vi "PSRR.vi"() -> ()   [LabVIEW 2020]
uses:
  pmbus_ltm4676a/controls/ltm4676a_config.ctl
  controls/psrr_nightwing_config.ctl
  controls/psrr_heatwave_config.ctl
  controls/psrr_scope_config.ctl
  controls/psrr_fgen_sweep_config.ctl
  <instrlib>/niDCPower/nidcpower.llb/niDCPower Source Mode.ctl
  <instrlib>/niDCPower/nidcpower.llb/niDCPower Output Function.ctl
  <instrlib>/niDCPower/nidcpower.llb/niDCPower Sense.ctl
  <instrlib>/niDCPower/nidcpower.llb/niDCPower Wait For Event - Event.ctl
  <instrlib>/niFgen/niFgen.llb/niFgen Output Mode.ctl
  <instrlib>/niScope/Controls/niScope vertical coupling.ctl
  <instrlib>/niScope/Controls/niScope trigger slope.ctl
  <instrlib>/niScope/Controls/niScope trigger coupling.ctl
  <instrlib>/niScope/Controls/niScope trigger source.ctl
  <instrlib>/niScope/Utility/niScope Get Channel Name From String.vi
  <instrlib>/niScope/Configure/Trigger/niScope Configure Trigger Edge.vi
panel:
  in  "App control":enum32{"Main", "Debug", "Ref"}(tab)
  in  "Calculation method":enum16{"RMS", "Peak-to-peak"}(ring)
  in  "Stop":bool
  in  "Step delay (ms)":u32=50
  in  "Continue sweep":bool
  in  "Step mode":enum16{"Timed", "User"}(ring)
  in  "Config control":T1(tab)
  in  "Source config":T2={"Source device name"="Nightwing", "Source device channel"="0", "Source device voltage (V)"=18.0, "Source current limit (A)"=6.0, "Channel setup time (s)"=0.5} {"Channel setup time (s)" format="%_4p"}
  in  "Load config":T3={"Load device name"="Heat-Wave", "Load device channel"="0", "Load device current (A)"=1.0, "Load voltage limit (V)"=6.0, "Channel setup time (s)"=0.5} {"Channel setup time (s)" format="%_4p"}
  in  "FGEN/sweep config":T4={"FGEN Resource Name"="Dev1", "Channel"="0", "Standard Waveform"=0, "Amplitude"=0.05, "Load impedance"=10000.0, "Sweep type"=1, "Points or Points/Decade"=10, "Start frequency"=10.0, "Stop frequency"=1000000.0} {"Load impedance" min=0.0 step=1000.0 format="%.2p"; "Stop frequency" min=0.0 step=1000.0 format="%.2p"; "Start frequency" min=0.0 step=1000.0 format="%.2p"; "Points or Points/Decade" min=1 step=1; "Sweep type" items=["Linear", "Logarithmic"]; "Amplitude" format="%.2p"; "Standard Waveform" items=["Sine", "Square", "Triangle", "Ramp Up", "Ramp Down", "DC", "Noise"]}
  in  "Scope config":T5={"Resource name"="Dev1", "Scope channel(s)"="0,1", "Probe Attenuation"=10.0, "Samples per cycle"=1000, "Cycles to acquire"=4} {"Cycles to acquire" min=1 step=1; "Probe Attenuation" format="%.1f"; "Samples per cycle" step=1000000}
  in  "LTM4676A Runtime Config":T6={"SDC config path"=path "C:/Users/Administrator/Documents/qkocian-sandbox/demos/argus-buck-demo/instrumentstudio/sdc/pmbus_ltm4676a.sdconfig", "Output setpoint (V)"=3.3, "Voltage margin (%)"=5.0, "Voltage warn limit (%)"=7.5, "Voltage fault limit (%)"=10.0, "Switching frequency (kHz)"=650} {"Switching frequency (kHz)" items=["250"=62440, "350"=64188, "425"=64338, "500"=64488, "575"=575, "650"=650, "750"=750, "1000"=1000]; "Voltage fault limit (%)" min=0.0 max=100.0 step=1.0 format="%.1g"; "Voltage warn limit (%)" min=0.0 max=100.0 step=1.0 format="%.1g"; "Voltage margin (%)" min=0.0 max=100.0 step=1.0 format="%.1g"; "Output setpoint (V)" min=0.5 max=5.5 step=0.1}
  out "Power Supply Rejection Ratio (dB)":cluster{dbl[], dbl[]}(graph) caption="Current (Amps) vs Voltage (Volts)"
  in  "Continue sweep (debug)":bool
  out "Output spectrum(s)":T7(graph)
  out "success?":bool
  in  "Use PMBus?":bool
  out "Input waveform(s)":waveform(dbl)[](graph)
  out "Filtered waveform(s)":waveform(dbl)[](graph) caption="Output waveform(s)"
  out "Detected frequencies":dbl[](array[numeric])
  out "Detected amplitudes":dbl[](array[numeric])
  out "Detected phases (deg)":dbl[](array[numeric])
  out "Actual sample rate":dbl=10000000.0 format="%#.2p"
  out "Actual record length":i32=1000
  out "Reqested sample rate":dbl
  out "Requested record length":i32
  out "Supply voltage":dbl[](array[numeric])
  out "Supply current":dbl[](array[numeric])
  out "Load voltage":dbl[](array[numeric])
  out "Load current":dbl[](array[numeric])
  out "Sweep values":dbl[](array[numeric]) format="%_6g"
  out "PSRR array":dbl[](array[numeric])
  # "(only for Step mode = Timed)"
  # "(only for Step mode = User)"
  # "(only for Step mode = User)"
  # "J2120A Information"
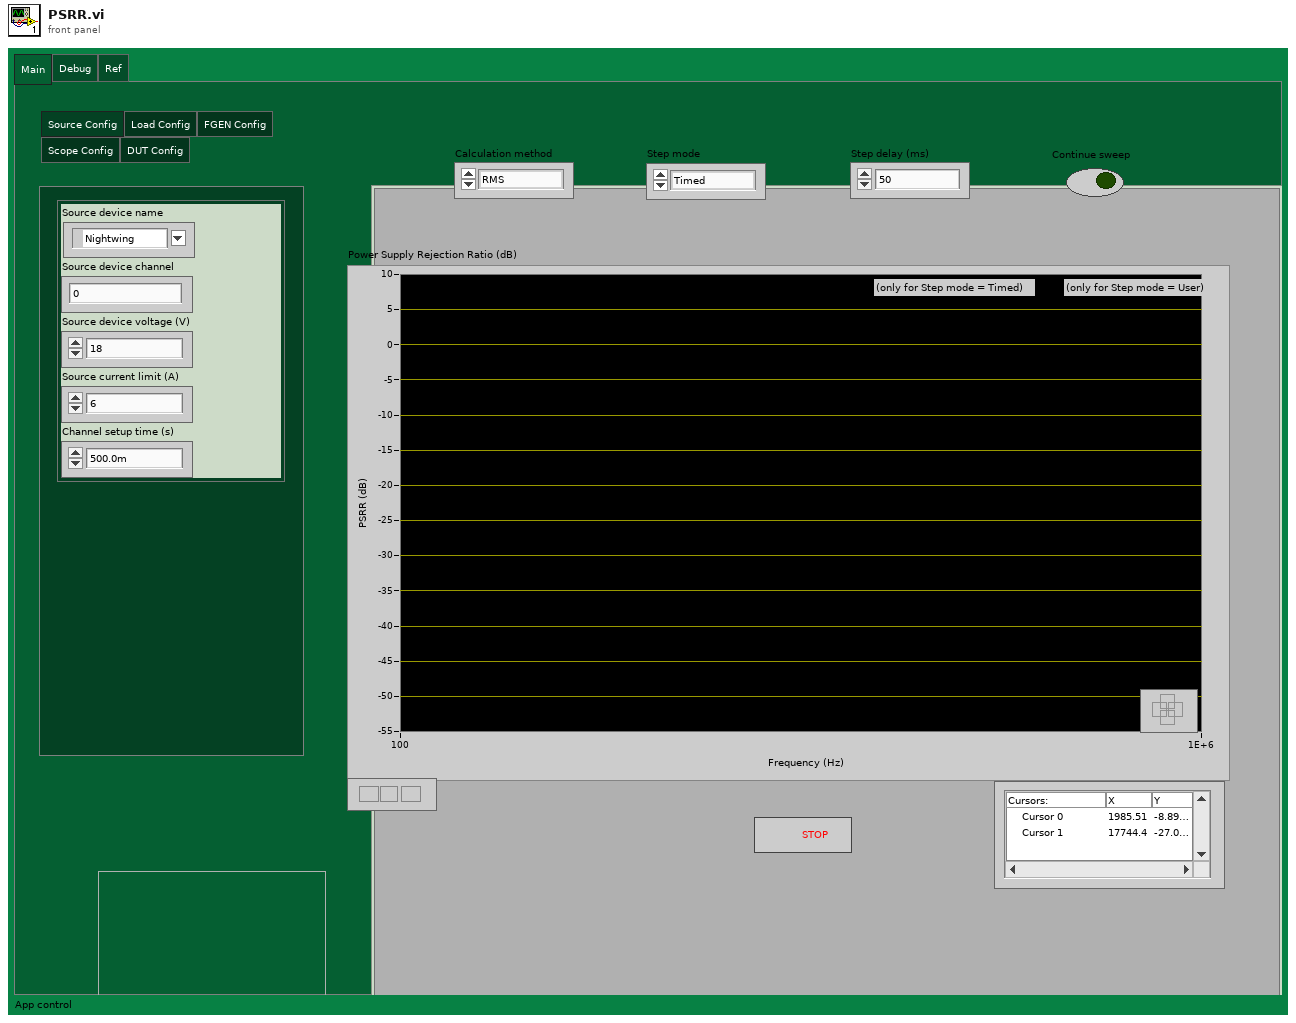
[diagram p1: front panel]
types:
  T1 = enum32{"Source Config", "Load Config", "FGEN Config", "Scope Config", "DUT Config"}
  T2 = typedef "psrr_nightwing_config.ctl" = cluster{"Source device name":refnum<k15>, "Source device channel":string, "Source device voltage (V)":dbl, "Source current limit (A)":dbl, "Channel setup time (s)":dbl}
  T3 = typedef "psrr_heatwave_config.ctl" = cluster{"Load device name":refnum<k15>, "Load device channel":string, "Load device current (A)":dbl, "Load voltage limit (V)":dbl, "Channel setup time (s)":dbl}
  T4 = typedef "psrr_fgen_sweep_config.ctl" = cluster{"FGEN Resource Name":refnum<k15>, "Channel":string, "Standard Waveform":u16, "Amplitude":dbl, "Load impedance":dbl, "Sweep type":u16, "Points or Points/Decade":u16, "Start frequency":dbl, "Stop frequency":dbl}
  T5 = typedef "psrr_scope_config.ctl" = cluster{"Resource name":refnum<k15>, "Scope channel(s)":string, "Probe Attenuation":dbl, "Samples per cycle":u32, "Cycles to acquire":u16}
  T6 = typedef "ltm4676a_config.ctl" = cluster{"SDC config path":path, "Output setpoint (V)":dbl, "Voltage margin (%)":dbl, "Voltage warn limit (%)":dbl, "Voltage fault limit (%)":dbl, "Switching frequency (kHz)":u16}
  T7 = cluster{"f0":dbl, "df":dbl, "dB Spectrum (Hann)":dbl[]}[]
  T8 = typedef "niDCPower Wait For Event - Event.ctl" = i32
  T9 = typedef "niDCPower Sense.ctl" = i32
  T10 = typedef "niDCPower Output Function.ctl" = i32
  T11 = typedef "niDCPower Source Mode.ctl" = i32
  T12 = typedef "niScope trigger source.ctl" = string
  T13 = typedef "niScope trigger coupling.ctl" = u16
  T14 = typedef "niScope trigger slope.ctl" = i32
  T15 = typedef "niScope vertical coupling.ctl" = i32
  T16 = typedef "niFgen Output Mode.ctl" = u32
  T17 = cluster{"Detected frequencies":dbl[], "Detected amplitudes":dbl[], "Detected phases (deg)":dbl[]}
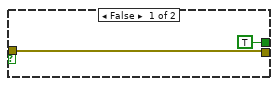
[diagram p2: hidden frame]
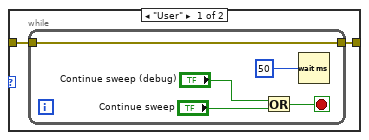
[diagram p4: hidden frame]
diagram:
  w8 = T8 1030 items=["Source Complete Event"=1030, "Measure Complete Event"=1031, "Sequence Iteration Complete Event"=1032, "Sequence Engine Done Event"=1033, "Pulse Complete Event"=1051, "Ready For Pulse Trigger Event"=1052] ("event")
  w31 = 1042 items=["Slow"=1041, "Normal"=1038, "Fast"=1039, "Custom"=1042] ("Source:Transient Response")
  w38 = T9 1008 items=["Local"=1008, "Remote"=1009] ("sense")
  w41 = 1026 items=["Automatically after Source Complete"=1025, "On Demand"=1026, "On Measure Trigger"=1027] ("Measurement:Advanced:Measure When")
  w50 = 1 items=["Off", "On"] ("Source:DC Voltage:Current Limit Autorange")
  w52 = T10 1006 items=["DC Voltage"=1006, "DC Current"=1007, "Pulse Voltage"=1049, "Pulse Current"=1050] ("output function")
  w55 = T11 1020 items=["Single Point"=1020, "Sequence"=1021] ("source mode")
  n1 = Unbundle By Name("Source config") -> ("Source device channel"=w1:string, "Source device name"=w29:refnum<k15>)
  n2 = call <instrlib>:"niDCPower Initialize With Independent Channels.vi"("resource name"=w29) -> ("error out"=w39:errorcluster, "instrument handle out"=w40:refnum<k15>)  [unwired: 9 in]
  n3 = call <instrlib>:"niDCPower Configure Sense.vi"("error in (no error)"=w39, "sense"=w38, "channel name"=w1, "instrument handle"=w40) -> ("error out"=w28:errorcluster, "instrument handle out"=w27:refnum<k15>)  [unwired: 6 in]
  n4 = call <instrlib>:"niDCPower Configure Source Mode With Channels.vi"("error in (no error)"=w28, "source mode"=w55, "channel name"=w1, "instrument handle"=w27) -> ("error out"=w54:errorcluster, "instrument handle out"=w53:refnum<k15>)  [unwired: 6 in]
  n5 = Unbundle By Name("Source config") -> ("Source device voltage (V)"=w13:dbl, "Source current limit (A)"=w14:dbl, "Channel setup time (s)"=w12:dbl)
  n6 = call <instrlib>:"niDCPower Configure Output Function.vi"("error in (no error)"=w54, "output function"=w52, "channel name"=w1, "instrument handle"=w53) -> ("error out"=w45:errorcluster, "instrument handle out"=w44:refnum<k15>)  [unwired: 6 in]
  n7 = call <instrlib>:"niDCPower Configure Voltage Level.vi"("error in (no error)"=w45, "voltage level"=w13, "channel name"=w1, "instrument handle"=w44) -> ("error out"=w42:errorcluster, "instrument handle out"=w43:refnum<k15>)  [unwired: 6 in]
  n8 = call <instrlib>:"niDCPower Configure Current Limit.vi"("error in (no error)"=w42, "current limit"=w14, "channel name"=w1, "instrument handle"=w43) -> ("error out"=w51:errorcluster, "instrument handle out"=w49:refnum<k15>)  [unwired: 6 in]
  n9 = property class="niDCPower"(reference=w49, error in=w51, "Active Channel"=w1, "Voltage Level Autorange"=w50, "Current Limit Autorange"=w50, "Source Delay"=w12, "Measure When"=w41) -> (reference out=w35:refnum<k15>, error out=w34:errorcluster)
  n10 = property class="niDCPower"(reference=w35, error in=w34, "Active Channel"=w1, "Transient Response"=w31, "Voltage GBW"=1000.0 ("Source:Custom Transient Response:Voltage:Gain Bandwidth"), "Voltage Compensation Freq"=1000.0 ("Source:Custom Transient Response:Voltage:Compensation Frequency"), "Voltage Pole-Zero Ratio"=1.0 ("Source:Custom Transient Response:Voltage:Pole-Zero Ratio"), "Current GBW"=1000000.0 ("Source:Custom Transient Response:Current:Gain Bandwidth")) -> (reference out=w33:refnum<k15>, error out=w32:errorcluster)
  n11 = call <instrlib>:"niDCPower Commit With Channels.vi"("error in (no error)"=w32, "channel name"=w1, "instrument handle"=w33) -> ("error out"=w36:errorcluster, "instrument handle out"=w37:refnum<k15>)  [unwired: 7 in]
  n12 = call <instrlib>:"niDCPower Initiate With Channels.vi"("error in (no error)"=w36, "channel name"=w1, "instrument handle"=w37) -> ("error out"=w9:errorcluster, "instrument handle out"=w10:refnum<k15>)  [unwired: 7 in]
  n13 = call <instrlib>:"niDCPower Wait For Event With Channels.vi"("error in (no error)"=w9, "event"=w8, "channel name"=w1, "instrument handle"=w10) -> ("error out"=w7:errorcluster, "instrument handle out"=w6:refnum<k15>)  [unwired: 6 in]
  n14 = call <instrlib>:"niDCPower Measure Multiple.vi"("error in (no error)"=w7, "channel name"=w1, "instrument handle"=w6) -> ("error out"=w5:errorcluster, "current measurements"=→"Supply current":dbl[], "voltage measurements"=→"Supply voltage":dbl[], "instrument handle out"=w4:refnum<k15>)  [unwired: 5 in]
  n15 = case shown="True" "Use PMBus?" {
    tunnel: [w57 w61] -> w26
    tunnel: w5 -> [w57 w60]
    tunnel: [TRUE ("success?") w58] -> w22
    frame False {
    }
    frame True {
      n16 = call "ltm4676a_set_runtime_config.vi"("LTM4676A Runtime Config"="LTM4676A Runtime Config", "error in (no error)"=w60) -> ("success?"=w58:bool, "error out"=w61:errorcluster)  [unwired: 1 out]
      "success?" <- w58
    }
  }
  n17 = case shown="True" w22 {
    tunnel: w26 -> [w62 w178]
    tunnel: [w62 w106] -> w11
    tunnel: w4 -> [w64 w74]
    tunnel: [w64 w72] -> w21
    tunnel: w1 -> [w63 w73]
    tunnel: [w63 w71] -> w20
    frame False {
    }
    frame True {
      w86 = T10 1007 items=["DC Voltage"=1006, "DC Current"=1007, "Pulse Voltage"=1049, "Pulse Current"=1050] ("output function")
      w87 = T11 1020 items=["Single Point"=1020, "Sequence"=1021] ("source mode")
      w89 = 1026 items=["Automatically after Source Complete"=1025, "On Demand"=1026, "On Measure Trigger"=1027] ("Measurement:Advanced:Measure When")
      w134 = 1 items=["None"=1, "Auto Trigger"=2] ("Triggering:Trigger Modifier")
      w141 = T13 1 items=["AC"=0, "DC"=1, "HF Reject"=3, "LF Reject"=4, "AC Plus HF Reject"=1001] ("trigger coupling")
      w142 = T14 0 items=["Positive", "Negative"] ("trigger slope")
      w145 = T15 0 items=["AC", "DC", "Ground"] ("vertical coupling")
      w148 = u32 0 items=["1 mega ohm"=0, "50 ohms"=2] ("input impedance")
      w159 = T16 0 items=["Standard Function", "Frequency List", "Arbitrary Waveform", "Arbitrary Sequence", "Script"] ("Output Mode (default: 0=Standard Function)")
      w90 = 1 items=["Off", "On"] ("Source:DC Current:Current Level Autorange")
      w181 = 1042 items=["Slow"=1041, "Normal"=1038, "Fast"=1039, "Custom"=1042] ("Source:Transient Response")
      w184 = T8 1030 items=["Source Complete Event"=1030, "Measure Complete Event"=1031, "Sequence Iteration Complete Event"=1032, "Sequence Engine Done Event"=1033, "Pulse Complete Event"=1051, "Ready For Pulse Trigger Event"=1052] ("event")
      w187 = T9 1009 items=["Local"=1008, "Remote"=1009] ("sense")
      n18 = Unbundle By Name("Load config") -> ("Load device channel"=w69:string, "Load device name"=w179:refnum<k15>)
      n19 = call <instrlib>:"niDCPower Initialize With Independent Channels.vi"("error in (no error)"=w178, "resource name"=w179) -> ("error out"=w189:errorcluster, "instrument handle out"=w188:refnum<k15>)  [unwired: 8 in]
      n20 = call <instrlib>:"niDCPower Configure Sense.vi"("error in (no error)"=w189, "sense"=w187, "channel name"=w69, "instrument handle"=w188) -> ("error out"=w93:errorcluster, "instrument handle out"=w96:refnum<k15>)  [unwired: 6 in]
      n21 = Unbundle By Name("Load config") -> ("Load device current (A)"=w88:dbl, "Load voltage limit (V)"=w65:dbl, "Channel setup time (s)"=w172:dbl)
      n22 = call <instrlib>:"niDCPower Configure Source Mode With Channels.vi"("error in (no error)"=w93, "source mode"=w87, "channel name"=w69, "instrument handle"=w96) -> ("error out"=w92:errorcluster, "instrument handle out"=w95:refnum<k15>)  [unwired: 6 in]
      n23 = call <instrlib>:"niDCPower Configure Output Function.vi"("error in (no error)"=w92, "output function"=w86, "channel name"=w69, "instrument handle"=w95) -> ("error out"=w91:errorcluster, "instrument handle out"=w94:refnum<k15>)  [unwired: 6 in]
      n24 = call <instrlib>:"niDCPower Configure Current Level.vi"("error in (no error)"=w91, "current level"=w88, "channel name"=w69, "instrument handle"=w94) -> ("error out"=w66:errorcluster, "instrument handle out"=w67:refnum<k15>)  [unwired: 6 in]
      n25 = property class="niDCPower"(reference=w67, error in=w66, "Active Channel"=w69, "Current Level Autorange"=w90, "Voltage Limit Range"=w65, "Source Delay"=w172, "Measure When"=w89) -> (reference out=w177:refnum<k15>, error out=w176:errorcluster)
      n26 = property class="niDCPower"(reference=w177, error in=w176, "Active Channel"=w69, "Transient Response"=w181, "Current GBW"=5000.0 ("Source:Custom Transient Response:Current:Gain Bandwidth"), "Current Compensation Freq"=1000.0 ("Source:Custom Transient Response:Current:Gain Bandwidth"), "Current Pole-Zero Ratio"=1.0 ("Source:Custom Transient Response:Current:Gain Bandwidth"), "Voltage GBW"=1000000.0 ("Source:Custom Transient Response:Voltage:Gain Bandwidth")) -> (reference out=w103:refnum<k15>, error out=w102:errorcluster)
      n27 = call <instrlib>:"niDCPower Commit With Channels.vi"("error in (no error)"=w102, "channel name"=w69, "instrument handle"=w103) -> ("error out"=w182:errorcluster, "instrument handle out"=w183:refnum<k15>)  [unwired: 7 in]
      n28 = call <instrlib>:"niDCPower Initiate With Channels.vi"("error in (no error)"=w182, "channel name"=w69, "instrument handle"=w183) -> ("error out"=w186:errorcluster, "instrument handle out"=w185:refnum<k15>)  [unwired: 7 in]
      n29 = call <instrlib>:"niDCPower Wait For Event With Channels.vi"("error in (no error)"=w186, "event"=w184, "channel name"=w69, "instrument handle"=w185) -> ("error out"=w100:errorcluster, "instrument handle out"=w101:refnum<k15>)  [unwired: 6 in]
      n30 = call <instrlib>:"niDCPower Measure Multiple.vi"("error in (no error)"=w100, "channel name"=w69, "instrument handle"=w101) -> ("error out"=w99:errorcluster, "current measurements"=→"Load current":dbl[], "voltage measurements"=→"Load voltage":dbl[], "instrument handle out"=w70:refnum<k15>)  [unwired: 5 in]
      n31 = Unbundle By Name("FGEN/sweep config") -> ("Sweep type"=w162:u16, "Points or Points/Decade"=w161:u16, "Start frequency"=w158:dbl, "Stop frequency"=w160:dbl, "Channel"=w79:string, "FGEN Resource Name"=w171:refnum<k15>)
      n32 = call "generateSweep.vi"("Sweep type"=w162, "Points or Points/Decade"=w161, "Start frequency"=w158, "Stop frequency"=w160) -> ("Sweep values"=w118:dbl[], "error out"=w132:errorcluster)  [unwired: 9 in, 1 out]
      "Sweep values" <- w118
      n33 = Merge Errors(w132, w99) -> (w133:errorcluster)
      n34 = call <instrlib>:"niFgen Initialize With Channels.vi"("error in (no error)"=w133, "Channel Name"=w79, "Resource Name"=w171) -> ("error out"=w167:errorcluster, "Instrument Handle Out"=w170:refnum<k15>)  [unwired: 7 in]
      n35 = Unbundle By Name("FGEN/sweep config") -> ("Start frequency"=w121:dbl, "Stop frequency"=w120:dbl)
      n36 = Unbundle By Name("FGEN/sweep config") -> ("Standard Waveform"=w157:u16, "Amplitude"=w156:dbl, "Load impedance"=w155:dbl)
      n37 = call <instrlib>:"niFgen Configure Output Mode.vi"("error in (no error)"=w167, "Output Mode (default: 0=Standard Function)"=w159, "Instrument Handle"=w170) -> ("error out"=w166:errorcluster, "Instrument Handle Out"=w169:refnum<k15>)  [unwired: 6 in]
      n38 = property on="Power Supply Rejection Ratio (dB)" class="XYGraph (strict)"("XScale.Minimum"=w121, "XScale.Maximum"=w120, "XScale.Mapping Mode"=u8 1 ("X Scale.Mapping Mode"), "XScale.ScaleFit"=u8 0 ("X Scale.Scale Fit")) -> ()  [unwired: 2 in, 2 out]
      n39 = call <instrlib>:"niFgen Configure Standard Waveform.vi"("Instrument Handle"=w169, "Channel Name"=w79, "Waveform"=w157, "Frequency"=0.0, "Amplitude"=w156, "error in (no error)"=w166) -> ("Instrument Handle Out"=w168:refnum<k15>, "error out"=w165:errorcluster)  [unwired: 8 in]
      n40 = property class="niFgen"(reference=w168, error in=w165, "Active Channel"=w79, "Load Impedance"=w155) -> (reference out=w164:refnum<k15>, error out=w163:errorcluster)
      n41 = call <instrlib>:"niFgen Initiate Generation.vi"("error in (no error)"=w163, "Instrument Handle"=w164) -> ("error out"=w131:errorcluster, "Instrument Handle Out"=w128:refnum<k15>)  [unwired: 8 in]
      n42 = Unbundle By Name("Scope config") -> ("Probe Attenuation"=w130:dbl, "Scope channel(s)"=w143:string, "Resource name"=w144:refnum<k15>)  [unwired: 1 out]
      n43 = call <instrlib>:"niScope Initialize With Options.vi"("resource name"=w144, "reset device"=FALSE, "error in"=w131) -> ("instrument handle"=w154:refnum<k15>, "error out"=w151:errorcluster)  [unwired: 11 in]
      n44 = local read "FGEN/sweep config"() -> (w129:T4)
      n45 = Unbundle By Name(w129) -> ("Stop frequency"=w76:dbl, "Amplitude"=w78:dbl)
      n46 = call-poly <instrlib>:"niScope Get Channel Name (Poly).vi"("instrument handle"=w154, "index"=w143, "error in"=w151) -> ("instrument handle out"=w153:refnum<k15>, "channel name"=w123:string, "error out"=w150:errorcluster)  [unwired: 10 in]
      n47 = call <instrlib>:"niScope Configure Vertical.vi"("instrument handle"=w153, "probe attenuation"=w130, "vertical coupling"=w145, "channels"=w123, "vertical range"=w78, "vertical offset"=0.0, "error in"=w150) -> ("instrument handle out"=w152:refnum<k15>, "error out"=w149:errorcluster)  [unwired: 7 in]
      n48 = Multiply(x=w76, y=2.0) -> (x*y=w77:dbl)
      n49 = call <instrlib>:"niScope Configure Chan Characteristics.vi"("instrument handle"=w152, "channels"=w123, "input impedance"=w148, "maximum input frequency"=w77, "error in"=w149) -> ("instrument handle out"=w138:refnum<k15>, "error out"=w137:errorcluster)  [unwired: 9 in]
      n50 = property on="Property Node" class="niScope"(reference=w138, error in=w137, "Trigger Modifier"=w134) -> (reference out=w136:refnum<k15>, error out=w135:errorcluster)
      n51 = Unbundle By Name("Scope config") -> ("Cycles to acquire"=w125:u16, "Samples per cycle"=w124:u32)
      n52 = call-poly <instrlib>:"niScope Configure Trigger (poly).vi"("instrument handle"=w136, "trigger slope"=w142, "trigger coupling"=w141, "trigger source"=T12 "0", "trigger level"=0.0, "error in"=w135) -> ("instrument handle out"=w127:refnum<k15>, "error out"=w85:errorcluster)  [unwired: 8 in]
      n53 = for {
        tunnel: w128 -> [w229]
        tunnel: w127 -> [w247]
        tunnel: w125 -> [w214]
        tunnel: w124 -> [w245]
        tunnel: w123 -> [w244]
        tunnel: w79 -> [w228]
        tunnel: [w228] -> _
        tunnel: [w244] -> _
        tunnel: w118 -> [w217] mode=indexing
        shift-right: [w224] -> w107
        shift-left: w85 -> [w196]
        tunnel: [w243] -> w104
        tunnel: [w240] -> w108
        shift-right: [w236] -> _
        shift-left: dbl[] [] -> [w239]
        shift-right: [w237] -> _
        shift-left: dbl[] [] -> [w238]
        tunnel: "Calculation method" -> [w222]
        shift-right: [w201] -> w72
        shift-left: w74 -> [w202]
        shift-right: [w200] -> w71
        shift-left: w73 -> [w200]
        shift-right: [w197] -> _
        shift-left: w70 -> [w199]
        shift-right: [w198] -> w68
        shift-left: w69 -> [w198]
        stop <- w225 stop-if-true
        n54 = call <instrlib>:"niDCPower Measure Multiple.vi"("error in (no error)"=w196, "channel name"=w200, "instrument handle"=w202) -> ("error out"=w195:errorcluster, "current measurements"=w192:dbl[], "voltage measurements"=w193:dbl[], "instrument handle out"=w201:refnum<k15>)  [unwired: 5 in]
        n55 = local write "Supply current"(w192) -> ()
        n56 = local write "Supply voltage"(w193) -> ()
        n57 = call <instrlib>:"niDCPower Measure Multiple.vi"("error in (no error)"=w195, "channel name"=w198, "instrument handle"=w199) -> ("error out"=w194:errorcluster, "current measurements"=w190:dbl[], "voltage measurements"=w191:dbl[], "instrument handle out"=w197:refnum<k15>)  [unwired: 5 in]
        n58 = local write "Load voltage"(w191) -> ()
        n59 = local write "Load current"(w190) -> ()
        n60 = call "setFgenFreqWait.vi"("error in (no error)"=w194, "Frequency"=w217, "Channel"=w228, "Instrument handle"=w229) -> ("error out"=w246:errorcluster, "Instrument handle out"=w240:refnum<k15>)  [unwired: 6 in]
        n61 = call "acquireConstantSamples.vi"("Instrument handle"=w247, "Channel(s)"=w244, "Cycles to acquire"=w214, "Samples/cycle"=w245, "Frequency"=w217, "error in (no error)"=w246) -> ("Waveform(s)"=w215:waveform(dbl)[], "Instrument handle out"=w220:refnum<k15>, "Requested record length"=→"Requested record length":i32, "Reqested sample rate"=→"Reqested sample rate":dbl, "Actual record length"=w206:i32, "Actual sample rate"=→"Actual sample rate":dbl, "error out"=w219:errorcluster)  [unwired: 7 in]
        "Input waveform(s)" <- w215
        "Actual record length" <- w206
        n62 = call "filterWfmsButterworthBandpass.vi"("Instrument handle"=w220, "Reset filters"=TRUE, "Q factor"=2, "F0"=w217, "Order"=2, "error in (no error)"=w219, "Time signal(s) in"=w215) -> ("Instrument handle out"=w212:refnum<k15>, "Filtered time signal(s)"=w208:waveform(dbl)[], "error out"=w211:errorcluster)  [unwired: 5 in, 1 out]
        n63 = Divide(x=w206, y=2) -> (x/y=w204:dbl)
        n64 = To Unsigned Long Integer(number=w204) -> (unsigned 32bit integer=w203:u32)
        n65 = call "lastNSampWfms.vi"("Time signal(s) in"=w208, "error in (no error)"=w211, "Samples"=w203, "Instrument handle"=w212) -> ("error out"=w209:errorcluster, "Instrument handle out"=w210:refnum<k15>, "Shifted time signal(s)"=w207:waveform(dbl)[])  [unwired: 5 in]
        "Filtered waveform(s)" <- w207
        n66 = call "calculatePsrrRawWfms.vi"("Time signal(s) in"=w207, "error in (no error)"=w209, "Calculation method"=w222, "Search frequency"=w217, "Instrument handle"=w210) -> ("error out"=w230:errorcluster, "Detected wfm parameters"=w234:T17, "PSRR"=w235:dbl, "Instrument handle out"=w243:refnum<k15>)  [unwired: 2 in, 1 out]
        n67 = Unbundle By Name(w234) -> ("Detected frequencies"=→"Detected frequencies":dbl[], "Detected amplitudes"=→"Detected amplitudes":dbl[], "Detected phases (deg)"=→"Detected phases (deg)":dbl[])
        n68 = Build Array (concatenate)(w238, w217) -> (w237:dbl[])
        n69 = Build Array (concatenate)(w239, w235) -> (w236:dbl[])
        "PSRR array" <- w236
        n70 = case shown="\"Timed\", Default" "Step mode" {
          tunnel: w230 -> [w249 w256]
          tunnel: [w248 w256] -> w224
          frame "User" {
            n71 = while {
              tunnel: w249 -> [w254]
              tunnel: [w254] -> w248
              stop <- w252 stop-if-true
              n72 = Or(x="Continue sweep (debug)", y="Continue sweep") -> (x .or. y?=w252:bool)
              n73 = Wait (ms)(milliseconds to wait=u32 50) -> ()  [unwired: 1 out]
            }
          }
          frame "Timed", Default {
            n74 = Wait (ms)(milliseconds to wait="Step delay (ms)") -> ()  [unwired: 1 out]
          }
        }
        n75 = Bundle(w237, w236) -> (→"Power Supply Rejection Ratio (dB)":cluster{dbl[], dbl[]})  [unwired: 1 in]
        n76 = Or(x=w224, y="Stop") -> (x .or. y?=w225:bool)
      }
      n77 = call <instrlib>:"niScope Close.vi"("instrument handle"=w104, "error in"=w107) -> ("error out"=w116:errorcluster)  [unwired: 13 in]
      n78 = call <instrlib>:"niFgen Abort Generation.vi"("error in (no error)"=w116, "Instrument Handle"=w108) -> ("error out"=w115:errorcluster, "Instrument Handle Out"=w114:refnum<k15>)  [unwired: 8 in]
      n79 = call <instrlib>:"niFgen Close.vi"("error in (no error)"=w115, "Instrument Handle"=w114) -> ("error out"=w117:errorcluster)  [unwired: 9 in]
      n80 = call <instrlib>:"niDCPower Configure Output Enabled.vi"("error in (no error)"=w117, "output enabled"=FALSE, "channel name"=w68, "instrument handle"=w70) -> ("error out"=w113:errorcluster, "instrument handle out"=w112:refnum<k15>)  [unwired: 6 in]
      n81 = call <instrlib>:"niDCPower Reset With Channels.vi"("error in (no error)"=w113, "channel name"=w68, "instrument handle"=w112) -> ("error out"=w110:errorcluster, "instrument handle out"=w111:refnum<k15>)  [unwired: 7 in]
      n82 = call <instrlib>:"niDCPower Close.vi"("error in (no error)"=w110, "instrument handle"=w111) -> ("error out"=w106:errorcluster)  [unwired: 9 in]
    }
  }
  n83 = call <instrlib>:"niDCPower Configure Output Enabled.vi"("error in (no error)"=w11, "output enabled"=FALSE, "channel name"=w20, "instrument handle"=w21) -> ("error out"=w23:errorcluster, "instrument handle out"=w24:refnum<k15>)  [unwired: 6 in]
  n84 = call <instrlib>:"niDCPower Reset With Channels.vi"("error in (no error)"=w23, "channel name"=w20, "instrument handle"=w24) -> ("error out"=w47:errorcluster, "instrument handle out"=w48:refnum<k15>)  [unwired: 7 in]
  n85 = call <instrlib>:"niDCPower Close.vi"("error in (no error)"=w47, "instrument handle"=w48) -> ("error out"=w46:errorcluster)  [unwired: 9 in]
  n86 = call <vilib>:"Simple Error Handler.vi"("error in (no error)"=w46) -> ()  [unwired: 4 in, 5 out]
